vi "Configure Multi Trip Line.vi"(0 "VISA resource name":refnum<visa-resource-name>, 1 "Batch Group Number  [/BT] (1)":i32=1 min=1 max=12, 2 "Group (1)":i32=1 min=1 max=12 step=1, 3 "Trip Line (1)":i32=1 min=1 max=4 step=1, 4 "Enable Trip Line (False)":bool, 5 "Display Position (50)":i32=50 min=0 max=100 step=1, 6 "Color":cluster{"R":i32, "G":i32, "B":i32} {"B" min=0 max=255 step=1; "G" min=0 max=255 step=1; "R" min=0 max=255 step=1}, 7 "error in (no error)":errorcluster, 9 "Line Width (1: Normal)":i32(ring)=1 items=["Thin", "Normal", "Thick"]) -> (20 "VISA resource name out":refnum<visa-resource-name>, 21 "Batch Group Number":i32, 22 "Group":i32, 23 "Trip Line":i32, 27 "error out":errorcluster)   [LabVIEW 2020, in "Yokogawa GX Series.lvlib"]
doc: "Sets the trip line for a display group. (/BT Option)\n\nCommand: SMltTripLine"
uses:
  <instrlib>/Yokogawa GX Series/Yokogawa GX Series.lvlib
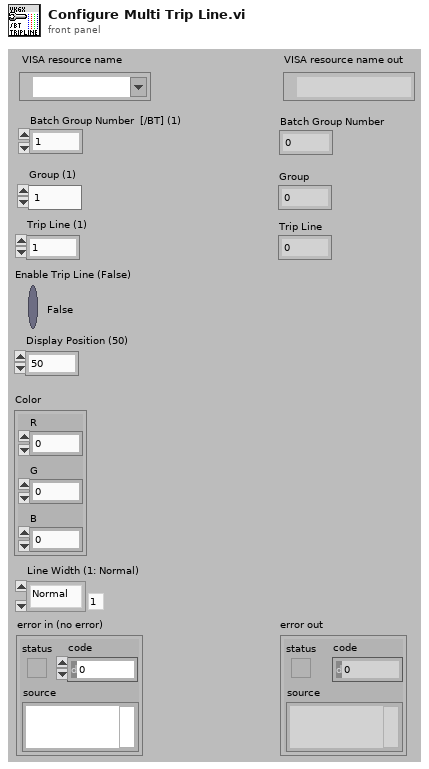
[diagram p1: front panel]
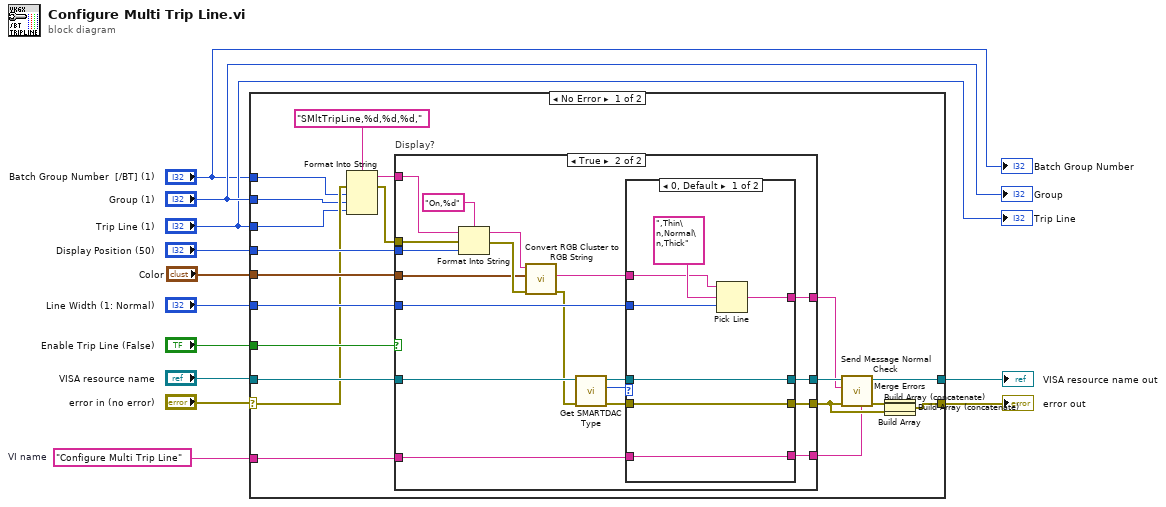
[diagram p0: block diagram]
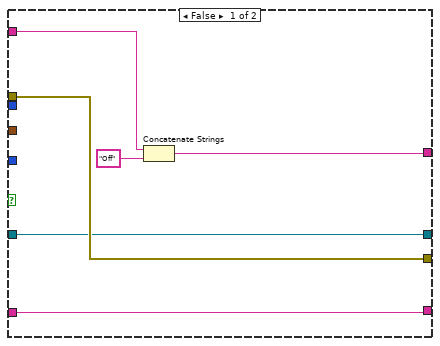
[diagram p2: hidden frame]
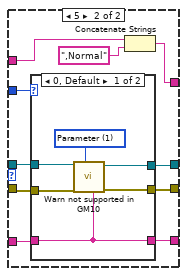
[diagram p3: hidden frame]
diagram:
  w10 = "Configure Multi Trip Line"  # VI name
  n1 = case shown="No Error" "error in (no error)" {
    selector: "error in (no error)" -> [w20 w87]
    tunnel: "Enable Trip Line (False)" -> [w35 _]
    tunnel: "Display Position (50)" -> [w34 _]
    tunnel: w10 -> [w26 _]
    tunnel: "Line Width (1: Normal)" -> [w33 _]
    tunnel: [w32 w88] -> w8
    tunnel: [w24 w87] -> w7
    tunnel: "Color" -> [w28 _]
    tunnel: "VISA resource name" -> [w21 w88]
    tunnel: "Group (1)" -> [w16 _]
    tunnel: "Trip Line (1)" -> [w17 _]
    tunnel: "Batch Group Number  [/BT] (1)" -> [w15 _]
    frame No Error {
      n2 = Format Into String(format string="SMltTripLine,%d,%d,%d,", error in=w20, w15, w16, w17) -> (resulting string=w29:string, error out=w30:errorcluster)  [unwired: 1 in]
      n3 = case "Display?" shown="True" w35 {
        tunnel: w30 -> [w41 w60]
        tunnel: [w41 w49] -> w23
        tunnel: w29 -> [w40 w58]
        tunnel: [w38 w54] -> w14
        tunnel: w34 -> [_ w59]
        tunnel: w33 -> [_ w55]
        tunnel: w28 -> [_ w56]
        tunnel: w21 -> [w37 w45]
        tunnel: [w37 w50] -> w27
        tunnel: w26 -> [w36 w48]
        tunnel: [w36 w47] -> w22
        frame False {
          n4 = Concatenate Strings(w40, "Off") -> (w38:string)
        }
        frame True {
          n5 = Format Into String(format string="On,%d", initial string=w58, error in=w60, w59) -> (resulting string=w51:string, error out=w57:errorcluster)
          n6 = call <instrlib>:"Convert RGB Cluster to RGB String.vi"("error in (no error)"=w57, "RGB"=w56, "Initial String"=w51) -> ("error out"=w44:errorcluster, "RGB String"=w52:string)  [unwired: 7 in]
          n7 = call <instrlib>:"Get SMARTDAC Type.vi"("error in (no error)"=w44, "VISA resource name"=w45) -> ("error out"=w43:errorcluster, "SMARTDAC+ Type"=w42:u16, "VISA resource name out"=w46:refnum<visa-resource-name>)  [unwired: 7 in]
          n8 = case shown="0, Default" w42 {
            tunnel: w55 -> [w67 w77]
            tunnel: [w65 w72] -> w54
            tunnel: w52 -> [w64 w73]
            tunnel: w46 -> [w62 w76]
            tunnel: [w62 w70] -> w50
            tunnel: w43 -> [w63 w75]
            tunnel: [w63 w69] -> w49
            tunnel: w48 -> [w61 w71]
            tunnel: [w61 w68] -> w47
            frame 0, Default {
              n9 = Pick Line(string ("")=w64, multi-line string=",Thin\n,Normal\n,Thick", line index=w67) -> (output string=w65:string)
            }
            frame 5 {
              n10 = case shown="0, Default" w77 {
                tunnel: w76 -> [w83 w86]
                tunnel: w75 -> [w78 w85]
                tunnel: w71 -> [w79 w84]
                tunnel: [w81 w86] -> w70
                tunnel: [w80 w85] -> w69
                tunnel: [w79 w84] -> w68
                frame 0, Default {
                  w82 = u16 1 items=["Command", "Parameter"] ("Kind (0: Command)")
                  n11 = call <instrlib>:"Warn not supported in GM10.vi"("Source (\"\")"=w79, "Kind (0: Command)"=w82, "error in (no error)"=w78, "VISA resource name"=w83) -> ("error out"=w80:errorcluster, "VISA resource name out"=w81:refnum<visa-resource-name>)  [unwired: 6 in]
                }
                frame 1 {
                }
              }
              n12 = Concatenate Strings(w73, ",Normal") -> (w72:string)
            }
          }
        }
      }
      n13 = call <instrlib>:"Send Message Normal Check.vi"("Source (\"\")"=w22, "error in (no error)"=w23, "Send Message (\"\")"=w14, "VISA resource name"=w27) -> ("error out"=w25:errorcluster, "VISA resource name out"=w32:refnum<visa-resource-name>)  [unwired: 2 in, 4 out]
      n14 = Build Array(w25, w23) -> (w19:errorcluster[])
      n15 = Build Array (concatenate)(w19) -> (w18:errorcluster[])
      n16 = Build Array (concatenate)(w18) -> (w13:errorcluster[])
      n17 = Merge Errors(w13) -> (w24:errorcluster)
    }
    frame Error {
    }
  }
  "error out" <- w7
  "VISA resource name out" <- w8
  "Group" <- "Group (1)"
  "Trip Line" <- "Trip Line (1)"
  "Batch Group Number" <- "Batch Group Number  [/BT] (1)"
